vi "Set Motor Output.vi"(8 "Speed Motor Outputs":dbl[](array[numeric]), 11 "Angle Motor Outputs":dbl[](array[numeric])) -> ()   [LabVIEW 2020]
uses:
  <vilib>/Rock Robotics/WPI/ThirdParty/Phoenix-LabVIEW/Motor Controller/Controls/CTRE_Phoenix_MotorControl_ControlMode.ctl
  <vilib>/Rock Robotics/WPI/ThirdParty/REV Robotics/REVLib/Typedef/Spark MAX Control Type.ctl
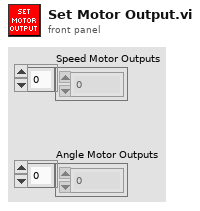
[diagram p1: front panel]
types:
  T1 = typedef "WPI_MotorControlDeviceRef.ctl" = cluster{"DeviceStatus":errorcluster, "Type":T2, "PWM":cluster{"PWM Channel":T3, "DeadBand":T4}, "CAN":cluster{"Device Number":u8, "SetOutput VI Ref":variant, "GetOutput VI Ref":variant, "Enable VI Ref":variant, "Disable VI Ref":variant, "Data":variant}, "Invert":bool, "DIO PWM":cluster{"PWM \"Enable\" Channel":T3, "DIOChannel":T5, "PWM Rate":dbl}}
  T2 = typedef "WPI_MotorControlType.ctl" = enum16{"PWM", "CAN", "DIO PWM"}
  T3 = typedef "FPGA_DIOPWMChannel.ctl" = enum8{"PWM 0", "PWM 1", "PWM 2", "PWM 3", "PWM 4", "PWM 5", "PWM 6", "PWM 7", "PWM 8", "PWM 9", "PWM MXP 0", "PWM MXP 1", "PWM MXP 2", "PWM MXP 3", "PWM MXP 4", "PWM MXP 5", "PWM MXP 6", "PWM MXP 7", "PWM MXP 8", "PWM MXP 9", "Invalid"}
  T4 = typedef "WPI_PWMDeadband.ctl" = cluster{"Name":string, "maxPositivePwm":i32, "minPositivePwm":i32, "centerPwm":i32, "maxNegativePwm":i32, "minNegativePwm":i32, "angularRange":u16}
  T5 = typedef "FPGA_DIOChannel.ctl" = enum8{"DIO 0", "DIO 1", "DIO 2", "DIO 3", "DIO 4", "DIO 5", "DIO 6", "DIO 7", "DIO 8", "DIO 9", "DIO MXP 0", "DIO MXP 1", "DIO MXP 2", "DIO MXP 3", "DIO MXP 4", "DIO MXP 5", "DIO MXP 6", "DIO MXP 7", "DIO MXP 8", "DIO MXP 9", "DIO MXP 10", "DIO MXP 11", "DIO MXP 12", "DIO MXP 13", "DIO MXP 14", "DIO MXP 15", "SPI Port CS1", "SPI Port CS2", "SPI Port CS3", "SPI Port MISO", "SPI Port MOSI", "Invalid"}
  T6 = typedef "CTRE_Phoenix_MotorControl_ControlMode.ctl" = u16
  T7 = typedef "Spark MAX Control Type.ctl" = enum16{"Percent VBus", "Voltage", "Velocity", "Position", "Smart Motion", "Current", "Smart Velocity"}
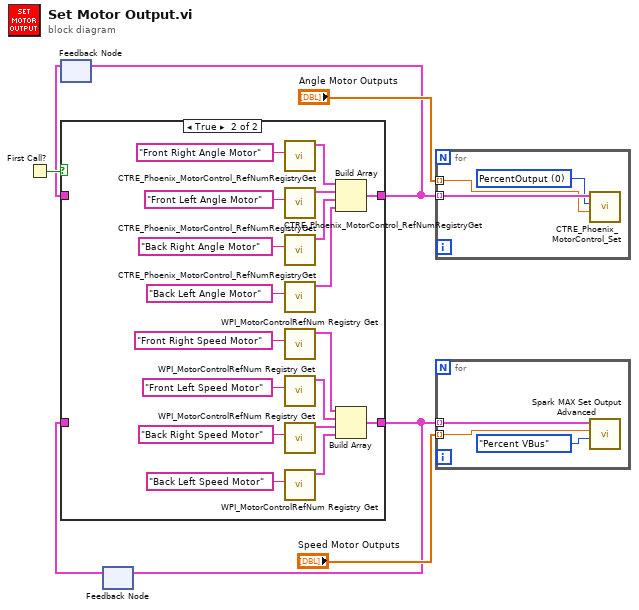
[diagram p0: block diagram]
diagram:
  n1 = First Call?() -> (First Call?: T/F=w5:bool)
  n2 = feedback #1() -> (w3:T1[])  [unwired: 1 in]
  n3 = feedback #2() -> (w1:T1[])  [unwired: 1 in]
  n4 = case shown="True" w5 {
    tunnel: [w9 w27] -> w4
    tunnel: w3 -> [w9 _]
    tunnel: [w8 w26] -> w2
    tunnel: w1 -> [w8 _]
    frame False {
    }
    frame True {
      n5 = call <vilib>:"CTRE_Phoenix_MotorControl_RefNumRegistryGet.vi"("refnum name"="Front Right Angle Motor") -> ("PhoenixMotorControlDevRef"=w20:T1)  [unwired: 9 in, 1 out]
      n6 = call <vilib>:"CTRE_Phoenix_MotorControl_RefNumRegistryGet.vi"("refnum name"="Front Left Angle Motor") -> ("PhoenixMotorControlDevRef"=w18:T1)  [unwired: 9 in, 1 out]
      n7 = call <vilib>:"CTRE_Phoenix_MotorControl_RefNumRegistryGet.vi"("refnum name"="Back Right Angle Motor") -> ("PhoenixMotorControlDevRef"=w17:T1)  [unwired: 9 in, 1 out]
      n8 = call <vilib>:"CTRE_Phoenix_MotorControl_RefNumRegistryGet.vi"("refnum name"="Back Left Angle Motor") -> ("PhoenixMotorControlDevRef"=w19:T1)  [unwired: 9 in, 1 out]
      n9 = call <vilib>:"WPI_MotorControlRefNum Registry Get.vi"("refnum name"="Front Right Speed Motor") -> ("MotorControlDevRef"=w16:T1)  [unwired: 9 in, 1 out]
      n10 = call <vilib>:"WPI_MotorControlRefNum Registry Get.vi"("refnum name"="Front Left Speed Motor") -> ("MotorControlDevRef"=w14:T1)  [unwired: 9 in, 1 out]
      n11 = call <vilib>:"WPI_MotorControlRefNum Registry Get.vi"("refnum name"="Back Right Speed Motor") -> ("MotorControlDevRef"=w12:T1)  [unwired: 9 in, 1 out]
      n12 = call <vilib>:"WPI_MotorControlRefNum Registry Get.vi"("refnum name"="Back Left Speed Motor") -> ("MotorControlDevRef"=w10:T1)  [unwired: 9 in, 1 out]
      n13 = Build Array(w20, w18, w17, w19) -> (w27:T1[])
      n14 = Build Array(w16, w14, w12, w10) -> (w26:T1[])
    }
  }
  n15 = feedback-in #1(w4) -> ()
  n16 = feedback-in #2(w2) -> ()
  n17 = for {
    tunnel: w4 -> [w30] mode=indexing
    tunnel: "Angle Motor Outputs" -> [w28] mode=indexing
    w29 = T6 0 items=["PercentOutput"=0, "Position"=1, "Velocity"=2, "Current"=3, "Follower"=5, "MotionProfile"=6, "MotionMagic"=7, "MotionProfileArc"=10, "Disabled"=15] ("Control Mode")
    n18 = call <vilib>:"CTRE_Phoenix_MotorControl_Set.vi"("Output"=w28, "Control Mode"=w29, "PhoenixMotorControlDevRef"=w30) -> ()  [unwired: 7 in, 2 out]
  }
  n19 = for {
    tunnel: w2 -> [w32] mode=indexing
    tunnel: "Speed Motor Outputs" -> [w31] mode=indexing
    n20 = call <vilib>:"Spark MAX Set Output Advanced.vi"("Control Mode"=Spark_MAX_Control_Type."Percent VBus", "Setpoint"=w31, "MotorControlDevRef"=w32) -> ()  [unwired: 7 in, 2 out]
  }
